vi "Get Window Bounds.vi"() -> ()   [LabVIEW 2022 SP3]
uses:
  <vilib>/Utility/miscctls.llb/LVRectTypeDef.ctl
  <vilib>/Utility/miscctls.llb/LVPointTypeDef.ctl
panel:
  out "Front Panel Window:Panel Bounds":T1
  in  "VI Name":string="SCM4 Interlock Network Client.vi"
  out "Front Panel Window:Window Bounds":T1
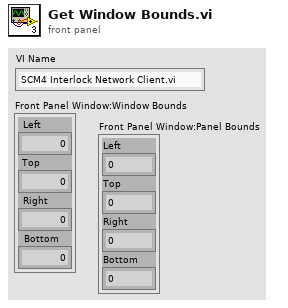
[diagram p1: front panel]
types:
  T1 = typedef "LVRectTypeDef.ctl" = cluster{"Left":i16, "Top":i16, "Right":i16, "Bottom":i16}
  T2 = typedef "LVPointTypeDef.ctl" = cluster{"Horizontal":i16, "Vertical":i16}
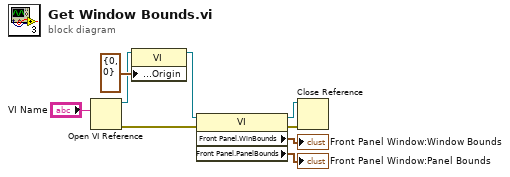
[diagram p0: block diagram]
diagram:
  n1 = Open VI Reference(vi path="VI Name") -> (vi reference=w3:refnum<vi>, error out=w7:errorcluster)  [unwired: 5 in]
  n2 = property class="VI"(reference=w3, "Front Panel Window:Origin"=T2 {"Horizontal"=0, "Vertical"=0}) -> (reference out=w2:refnum<vi>)  [unwired: 1 in, 1 out]
  n3 = property class="VI"(reference=w2, error in=w7) -> (reference out=w1:refnum<vi>, error out=w8:errorcluster, "Front Panel.WinBounds"=→"Front Panel Window:Window Bounds":T1, "Front Panel.PanelBounds"=→"Front Panel Window:Panel Bounds":T1)
  n4 = Close Reference(reference=w1, error in (no error)=w8) -> ()  [unwired: 1 out]
